vi "ClearTCPConnectionClosed.vi"(8 "error in (no error)":errorcluster) -> (0 "error out":errorcluster, 3 "TCP Closed?":bool)   [LabVIEW 2013]
uses:
  <vilib>/Utility/error.llb/DialogType.ctl
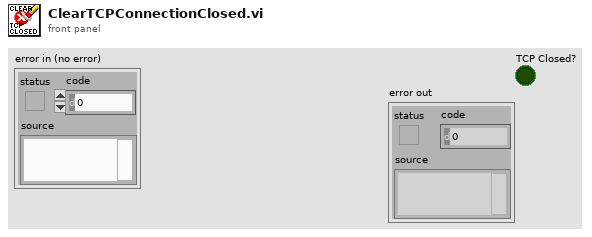
[diagram p1: front panel]
types:
  T1 = typedef "DialogType.ctl" = u16
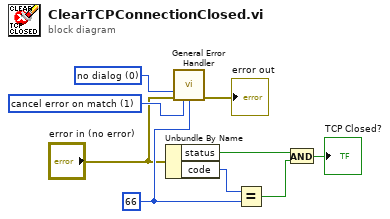
[diagram p0: block diagram]
diagram:
  w7 = 66 ("[exception code]")
  w8 = 1 items=["no exception", "cancel error on match", "set error on match"] ("[exception action] (none:0)")
  w9 = T1 0 items=["no dialog", "OK message", "continue or stop message", "OK message + warnings", "continue/stop + warnings"] ("type of dialog (OK msg:1)")
  n1 = Unbundle By Name("error in (no error)") -> ("status"=w4:bool, "code"=w5:i32)
  n2 = call <vilib>:"General Error Handler.vi"("type of dialog (OK msg:1)"=w9, "error in (no error)"="error in (no error)", "[exception action] (none:0)"=w8, "[exception code]"=w7) -> ("error out"=→"error out":errorcluster)  [unwired: 7 in, 4 out]
  n3 = Equal?(x=w5, y=w7) -> (x = y?=w3:bool)
  n4 = And(x=w4, y=w3) -> (x .and. y?=→"TCP Closed?":bool)
